vi "Save Info.vi"(7 "Overwrite? (T)":bool=TRUE, 8 "error in":errorcluster, 10 "filename":path, 11 "info data":string) -> (0 "error out":errorcluster)   [LabVIEW 2019, in "infolib.lvlib"]
doc: "Writes info string to a file. Extension of the file '.info' is added if missing."
uses:
  infolib.lvlib
  <vilib>/Utility/error.llb/Error Cluster From Error Code.vi
  <vilib>/ErrorRing/Error Ring.xnode
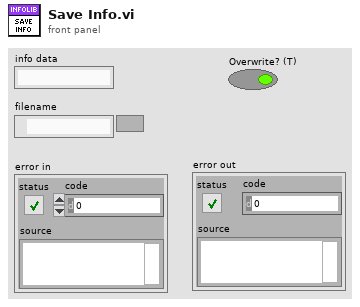
[diagram p1: front panel]
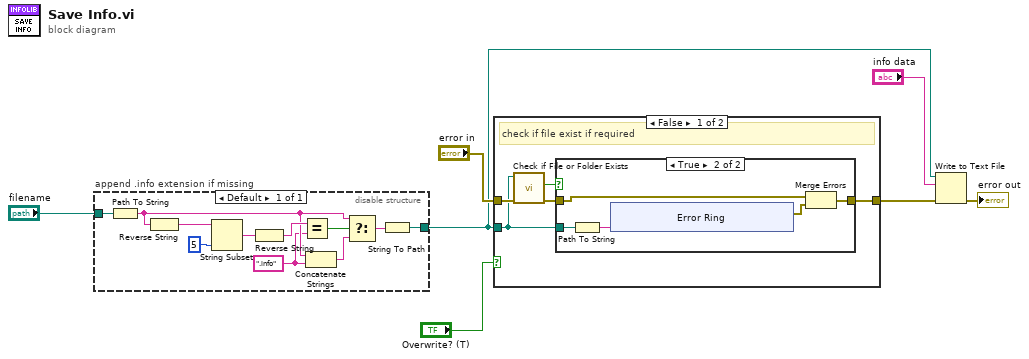
[diagram p0: block diagram]
diagram:
  n1 = disable-structure "append .info extension if missing" shown="Default" {
    disable-tunnel: "filename" -> [w18]
    disable-tunnel: [w8] -> w1
    frame Enabled {
      w11 = ".info" ("y")
      n2 = Path To String(path=w18) -> (string=w12:string)
      n3 = Reverse String(1:w12) -> (0:w17:string)
      n4 = String Subset(string=w17, length (rest)=5 ("length (rest)")) -> (substring=w16:string)  [unwired: 1 in]
      n5 = Reverse String(1:w16) -> (0:w14:string)
      n6 = Equal?(x=w14, y=w11) -> (x = y?=w13:bool)
      n7 = Concatenate Strings(w12, w11) -> (w10:string)
      n8 = Select(t=w12, s=w13, f=w10) -> (s? t:f=w9:string)
      n9 = String To Path(string=w9) -> (path=w8:path)
    }
  }
  n10 = case shown="False" "Overwrite? (T)" {
    tunnel: w1 -> [w19 _]
    tunnel: [w21 w37] -> w3
    tunnel: "error in" -> [w20 w37]
    frame False {
      # "check if file exist if required"
      n11 = call <vilib>:"Check if File or Folder Exists.vi"("error in (no error)"=w20, "path"=w19) -> ("error out"=w22:errorcluster, "file or folder exists?"=w23:bool)  [unwired: 7 in, 1 out]
      n12 = case shown="True" w23 {
        tunnel: w22 -> [w24 w29]
        tunnel: [w24 w27] -> w21
        tunnel: w19 -> [_ w25]
        frame False {
        }
        frame True {
          n13 = Path To String(path=w25) -> (string=w26:string)
          n14 = xnode "Error Ring"("parameter 0"=w26) -> ("error out"=w28:errorcluster)
          n15 = Merge Errors(w29, w28) -> (w27:errorcluster)
        }
      }
    }
    frame True {
    }
  }
  n16 = Write to Text File(file (use dialog)=w1, text="info data", error in=w3) -> (error out=→"error out":errorcluster)  [unwired: 1 in, 2 out]
